vi "Test3.vi"   [LabVIEW 2024]
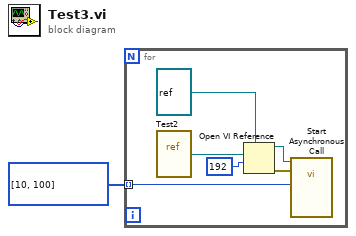
[diagram p0: block diagram]
diagram:
  n1 = for {
    tunnel: u32[] [10, 100] -> [w4] mode=indexing
    n2 = vi-ref "Test2.vi"() -> (w7:refnum<vi>)
    n3 = Open VI Reference(type specifier VI Refnum (for type only)=refnum<vi> refnum ("vi reference"), vi path=w7, options=192) -> (vi reference=w2:refnum<vi>, error out=w5:errorcluster)  [unwired: 3 in]
    n4 = call-by-ref "Start Asynchronous Call"(reference=w2, error in=w5, "millisecond multiple"=w4) -> ()  [unwired: 11 in, 2 out]
  }
